vi "Write TDMS-Data.vi"(8 "error in (no error)":errorcluster, 10 "TDMS-Data":refnum<class "TDMS-Data.lvclass">, 11 "Update TDMS-Data Msg in":refnum<class "Update TDMS-Data Msg.lvclass">) -> (0 "error out":errorcluster, 3 "Update TDMS-Data Msg out":refnum<class "Update TDMS-Data Msg.lvclass">)   [LabVIEW 2016, in "BNT_TDMS.lvlib" / "Update TDMS-Data Msg.lvclass"]
uses:
  Update TDMS-Data Msg.lvclass
  TDMSData/TDMS-Data.lvclass
  Update TDMS-Data Msg.lvclass/Update TDMS-Data Msg.ctl
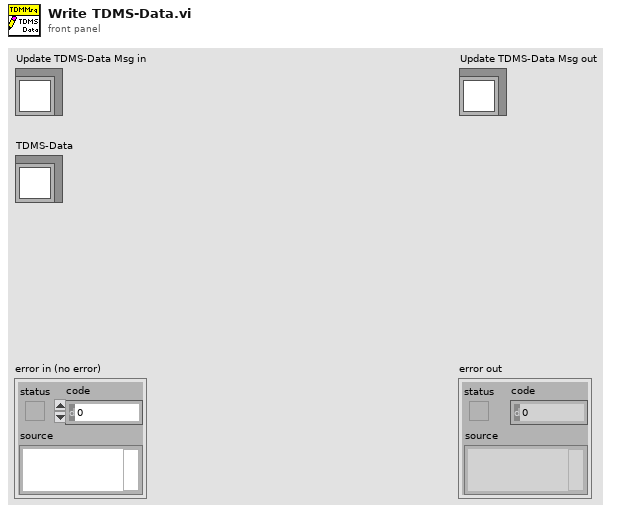
[diagram p1: front panel]
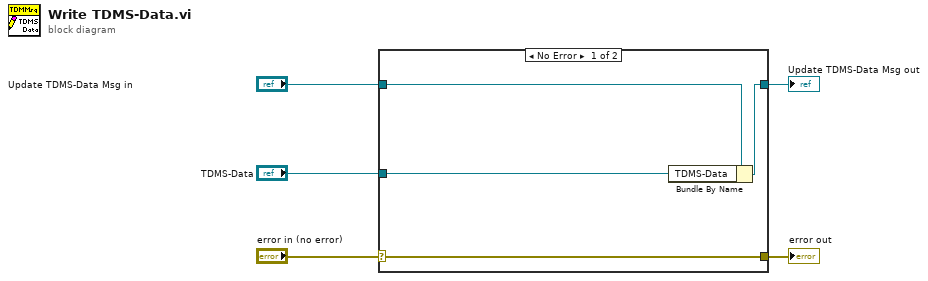
[diagram p0: block diagram]
diagram:
  n1 = case shown="No Error" "error in (no error)" {
    selector: "error in (no error)" -> [w9 w10]
    tunnel: [w9 w10] -> w4
    tunnel: [w7 w11] -> w2
    tunnel: "Update TDMS-Data Msg in" -> [w8 w11]
    tunnel: "TDMS-Data" -> [w6 _]
    frame No Error {
      n2 = Bundle By Name(cluster=w8, "TDMS-Data"=w6) -> (w7:refnum<class "Update TDMS-Data Msg.lvclass">)
    }
    frame Error {
    }
  }
  "error out" <- w4
  "Update TDMS-Data Msg out" <- w2
